vi "shippingWithInsertSublot.vi"() -> ()   [LabVIEW 2012]
uses:
  <vilib>/Utility/NIReport.llb/NI_report.lvclass
panel:
  out "error out 4":errorcluster
  out "String 3":string
  out "String 2":string
  out "appended path":path
  out "size(s)":i32
  out "error out":errorcluster
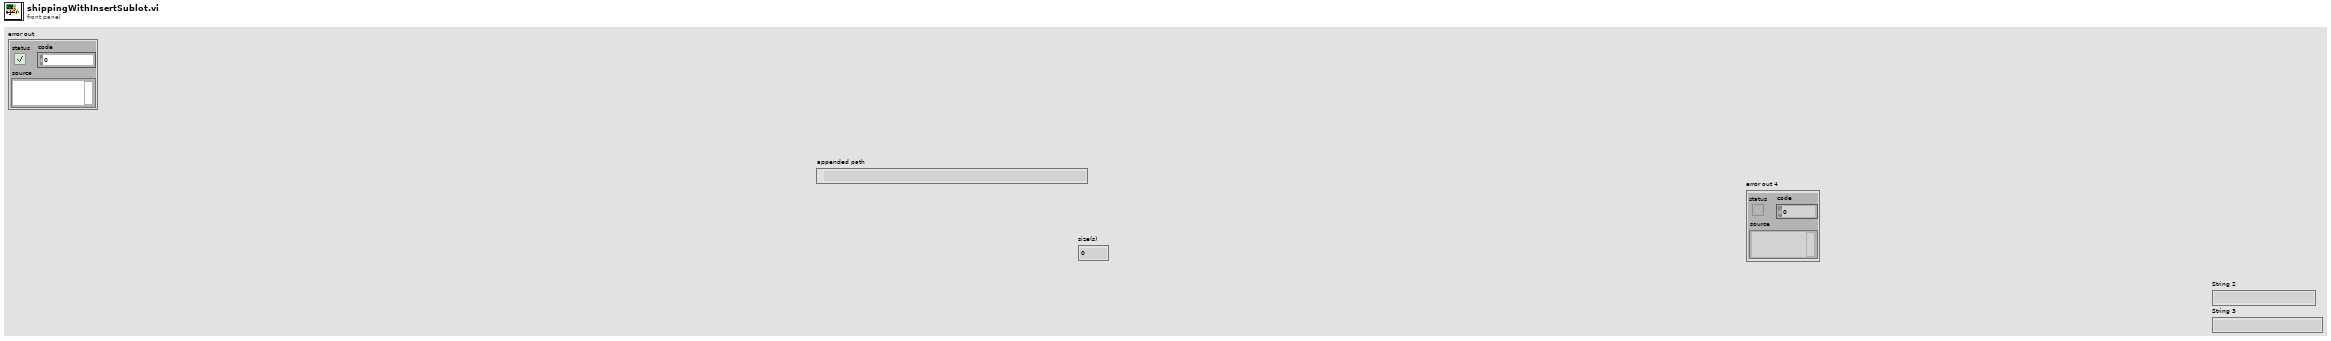
[diagram p1: front panel]
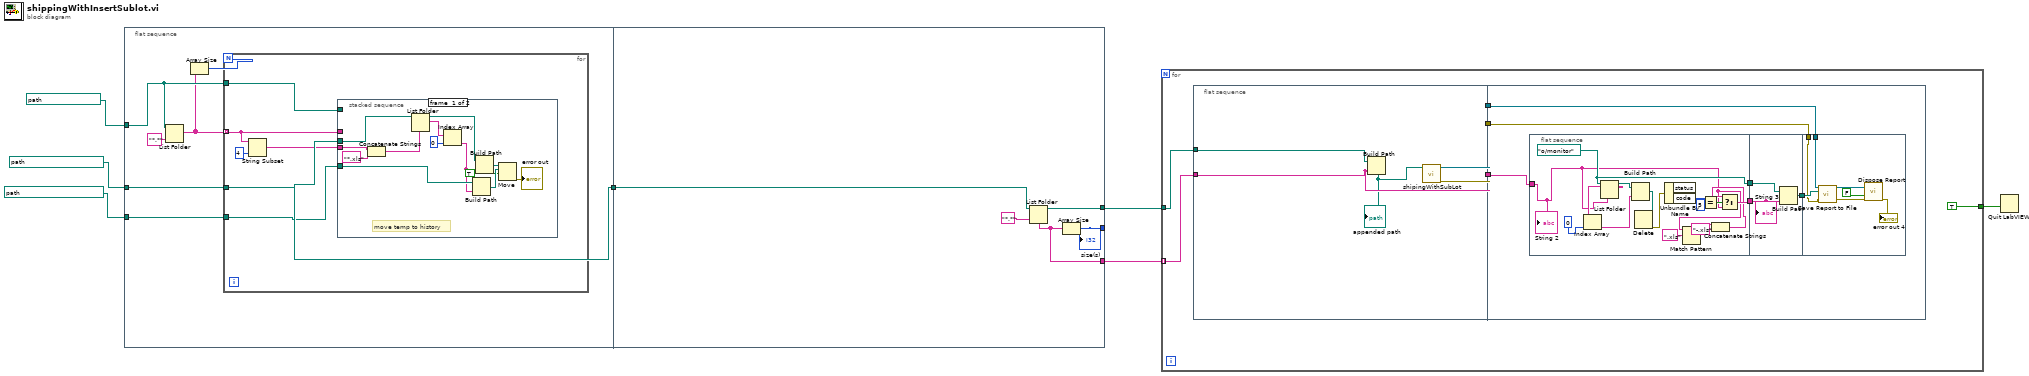
[diagram p0: block diagram]
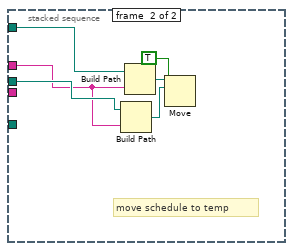
[diagram p2: hidden frame]
diagram:
  n1 = flat-sequence {
    tunnel: path "o:/monitor/回貨明細/temp" ("path") -> [w10]
    tunnel: [w10] -> w7
    tunnel: path "o:/monitor/回貨明細" ("path") -> [w12]
    tunnel: path "o:/monitor/回貨明細/history" ("path") -> [w11]
    tunnel: w7 -> [w42]
    tunnel: [w41] -> _
    tunnel: [w40] -> w2
    tunnel: [w39] -> w3
    frame #0 {
      n2 = List Folder(path=w12, pattern="*.*") -> (filenames=w8:string[])  [unwired: 2 in, 3 out]
      n3 = Array Size(array=w8) -> (size(s)=w9:i32)
      n4 = for {
        N: w9 -> [_]
        tunnel: w12 -> [w19]
        tunnel: w11 -> [w18]
        tunnel: w10 -> [w17]
        tunnel: w8 -> [w14] mode=indexing
        n5 = String Subset(string=w14, length (rest)=4 ("length (rest)")) -> (substring=w15:string)  [unwired: 1 in]
        n6 = stacked-sequence {
          tunnel: w17 -> [w28 w35]
          tunnel: w18 -> [w31 _]
          tunnel: w19 -> [_ w36]
          tunnel: w15 -> [w23 _]
          tunnel: w14 -> [_ w33]
          frame #0 {
            # "move temp to history"
            n7 = Concatenate Strings(w23, "*.xls" ("pattern")) -> (w21:string)
            n8 = List Folder(path=w28, pattern=w21) -> (path out=w27:path, filenames=w26:string[])  [unwired: 2 in, 2 out]
            n9 = Index Array(array=w26, index=0) -> (element=w24:string)
            n10 = Build Path(base path=w31, name or relative path=w24) -> (appended path=w30:path)
            n11 = Build Path(base path=w27, name or relative path=w24) -> (appended path=w32:path)
            n12 = Move(source path=w32, 9:TRUE ("overwrite (F)"), 10:w30) -> (error out=→"error out":errorcluster)  [unwired: 2 in, 2 out]
          }
          frame #1 {
            # "move schedule to temp"
            n13 = Build Path(base path=w35, name or relative path=w33) -> (appended path=w37:path)
            n14 = Build Path(base path=w36, name or relative path=w33) -> (appended path=w38:path)
            n15 = Move(source path=w38, 9:TRUE ("overwrite (F)"), 10:w37) -> ()  [unwired: 2 in, 3 out]
          }
        }
      }
    }
    frame #1 {
      n16 = List Folder(path=w42, pattern="*.*") -> (path out=w40:path, filenames=w39:string[])  [unwired: 2 in, 2 out]
      n17 = Array Size(array=w39) -> (size(s)=w41:i32)
      "size(s)" <- w41
    }
  }
  n18 = for {
    tunnel: [w48] -> _ mode=indexing
    tunnel: w3 -> [w48] mode=indexing
    tunnel: w2 -> [w49]
    tunnel: [TRUE] -> w1
    n19 = flat-sequence {
      tunnel: w49 -> [w54]
      tunnel: w48 -> [w53]
      tunnel: [w53] -> w47
      tunnel: [w51] -> w46
      tunnel: [w50] -> w45
      tunnel: w47 -> [w57]
      tunnel: w46 -> [w56]
      tunnel: w45 -> [w55]
      frame #0 {
        n20 = Build Path(base path=w54, name or relative path=w53) -> (appended path=w52:path)
        "appended path" <- w52
        n21 = call "shipingWithSubLot.vi"("template (empty)"=w52) -> ("error out"=w50:errorcluster, "report out"=w51:refnum<class "NI_report.lvclass">)  [unwired: 9 in]
      }
      frame #1 {
        n22 = flat-sequence {
          tunnel: [w62] -> w60
          tunnel: [w64] -> w59
          tunnel: w57 -> [w61]
          tunnel: w60 -> [w79]
          tunnel: w59 -> [w78]
          tunnel: [w77] -> w58
          tunnel: w58 -> [w82]
          tunnel: w56 -> [w81]
          tunnel: w55 -> [w80]
          frame #0 {
            w62 = path "o:/monitor" ("base path")
            n23 = List Folder(path=w62, pattern=w61) -> (path out=w74:path, filenames=w76:string[])  [unwired: 2 in, 2 out]
            n24 = Index Array(array=w76, index=0) -> (element=w73:string)
            n25 = Build Path(base path=w74, name or relative path=w73) -> (appended path=w72:path)
            n26 = Delete(path (use dialog)=w72) -> (error out=w71:errorcluster)  [unwired: 4 in, 2 out]
            n27 = Unbundle By Name(w71) -> ("code"=w70:i32)  [unwired: 1 out]
            n28 = Match Pattern(string=w61, regular expression=".xls") -> (match substring=w66:string)  [unwired: 1 in, 3 out]
            n29 = Equal?(x=w70, y=5) -> (x = y?=w68:bool)
            n30 = Concatenate Strings(w66, "-.xls" ("string")) -> (w63:string)
            n31 = Select(t=w63, s=w68, f=w61) -> (s? t:f=w64:string)
            "String 2" <- w61
          }
          frame #1 {
            n32 = Build Path(base path=w79, name or relative path=w78) -> (appended path=w77:path)
            "String 3" <- w78
          }
          frame #2 {
            n33 = call-dynamic "Save Report to File.vi"("report in"=w81, "report file path"=w82, "error in (no error)"=w80) -> ("report out"=w83:refnum<class "NI_report.lvclass">, "error out"=w84:errorcluster)  [unwired: 11 in]
            n34 = call-dynamic "Dispose Report.vi"("report in"=w83, "save changes? (F)"=FALSE, "error in (no error)"=w84) -> ("error out"=→"error out 4":errorcluster)  [unwired: 12 in]
          }
        }
      }
    }
  }
  n35 = Quit LabVIEW(quit? (T)=w1) -> ()
